vi "blackman_window.vi"() -> ()   [LabVIEW 2021]
uses:
  <vilib>/Analysis/4window.llb/Blackman-Harris Window (DBL).vi
  <vilib>/Analysis/4window.llb/AllCosWindow (DBL).vi
  <vilib>/Analysis/NI_AALPro.lvlib
panel:
  out "Init Data Out":fxp<+,16,0>[](array[numeric])
  out "Waveform Graph":dbl[](graph)
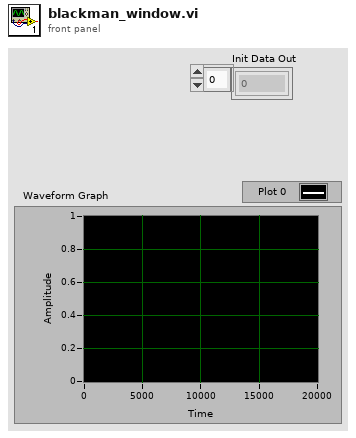
[diagram p1: front panel]
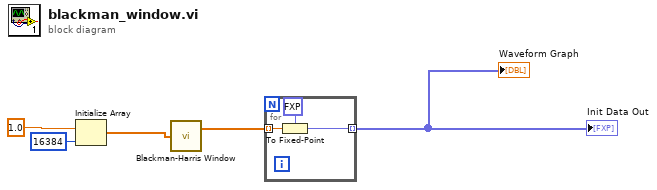
[diagram p0: block diagram]
diagram:
  n1 = Initialize Array(1.0 ("element"), 16384 ("dimension size")) -> (w3:dbl[])
  n2 = call-poly <vilib>:"Blackman-Harris Window.vi"("X"=w3) -> ("Windowed X"=w2:dbl[])  [unwired: 1 out]
  n3 = for {
    tunnel: w2 -> [w8] mode=indexing
    tunnel: [w7] -> w1 mode=indexing
    n4 = To Fixed-Point(fixed-point type=fxp<+,16,0> 0.0, number=w8) -> (fixed-point=w7:fxp<+,16,0>)
  }
  "Waveform Graph" <- w1
  "Init Data Out" <- w1
